vi "Main.InitializeXNET.vi"(7 "Name":string, 8 "error in (no error)":errorcluster, 10 "Data Settings":T12 {"MonitorTool"."Data"."Outgoing"."Trigger.Refs"."Data Reference" format="%.0x"; "MonitorTool"."Data"."Outgoing"."Disable.Refs"."Data Reference" format="%.0x"; "MonitorTool"."Data"."Outgoing"."Data.Refs"."Data Reference" format="%.0x"; "MonitorTool"."Data"."Incoming"."Timing.Refs"."Data Reference" format="%.0x"; "MonitorTool"."Data"."Incoming"."Data.Refs"."Data Reference" format="%.0x"; "MonitorTool"."Network"."Name" format="%.0x"; "SimNodes"."DTCs"."DM1 Ref"."Data Reference" format="%.0x"; "SimNodes"."DTCs"."DM1 Enable Ref"."Data Reference" format="%.0x"; "SimNodes"."DTCs"."DM2 Ref"."Data Reference" format="%.0x"; "SimNodes"."DTCs"."DM2 Enable Ref"."Data Reference" format="%.0x"; "SimNodes"."Network"."Name" format="%.0x"}, 11 "XNET Settings":T2 {"Termination" items=["Off", "On"]}) -> (0 "error out":errorcluster, 3 "Protocol App":T1={"XNET Settings"={"Database"="", "Cluster"="", "Port"="", "Baud rate [Bd]"=0, "Termination"=0, "Incoming Rate"=0, "Outcoming Rate"=1, "Write Decimation"=1}, "Data"=[], "DTCs"=[], "Sim Addresses LUT"=variant, "Data Table LUT"=variant, "MonitorTool.Network"={"Address"=0, "Name"=0}, "Name"=""} {"MonitorTool.Network"."Name" format="%.0x"; "DTCs"."Data"."DM1 Ref"."Data Reference" format="%.0x"; "DTCs"."Data"."DM1 Enable Ref"."Data Reference" format="%.0x"; "DTCs"."Data"."DM2 Ref"."Data Reference" format="%.0x"; "DTCs"."Data"."DM2 Enable Ref"."Data Reference" format="%.0x"; "Data"."Trigger.Refs"."Data Reference" format="%.0x"; "Data"."Disable.Refs"."Data Reference" format="%.0x"; "Data"."Timing.Refs"."Data Reference" format="%.0x"; "Data"."Network"."Name" format="%.0x"; "Data"."IncomingRefs"."Data Reference" format="%.0x"; "Data"."OutgoingRefs"."Data Reference" format="%.0x"; "XNET Settings"."Termination" items=["Off", "On"]})   [LabVIEW 2015, in "J1939 Addon Engine.lvlib"]
uses:
  J1939 Addon Engine.lvlib
  Shared/Types/XNET Settings.ctl
  Shared/Types/Compiled.Node Settings.ctl
  Shared/Types/Compiled Monitor Tool Settings.ctl
  Shared/Types/Monitor Settings.ctl
  Shared/Types/Device Settings.ctl
  Shared/Types/Incoming Settings.ctl
  Shared/Types/Frame Settings.ctl
  Shared/Types/Outgoing Event Trigger Types.ctl
  <vilib>/NI Veristand/Custom Device API/Block Data Reference.ctl
  <vilib>/NI Veristand/Custom Device API/Data Reference.ctl
  Shared/Types/Outgoing Settings.ctl
  Shared/Types/Complied Simulated Device Settings.ctl
  Shared/Types/Compiled Simulated Settings.ctl
  Types/Protocol.App Settings.ctl
  Types/Protocol.XNET Refs.ctl
  Types/Main.Outgoing.Frame.Settings.ctl
  Types/Engine.DTC Settings.ctl
  Types/Engine.DTC FIFOs.ctl
  Types/Engine.Node DTC Settings.ctl
  Shared/J1939 Addon Shared.lvlib
  <vilib>/NI VeriStand/Custom Device API/Custom Device API.lvlib
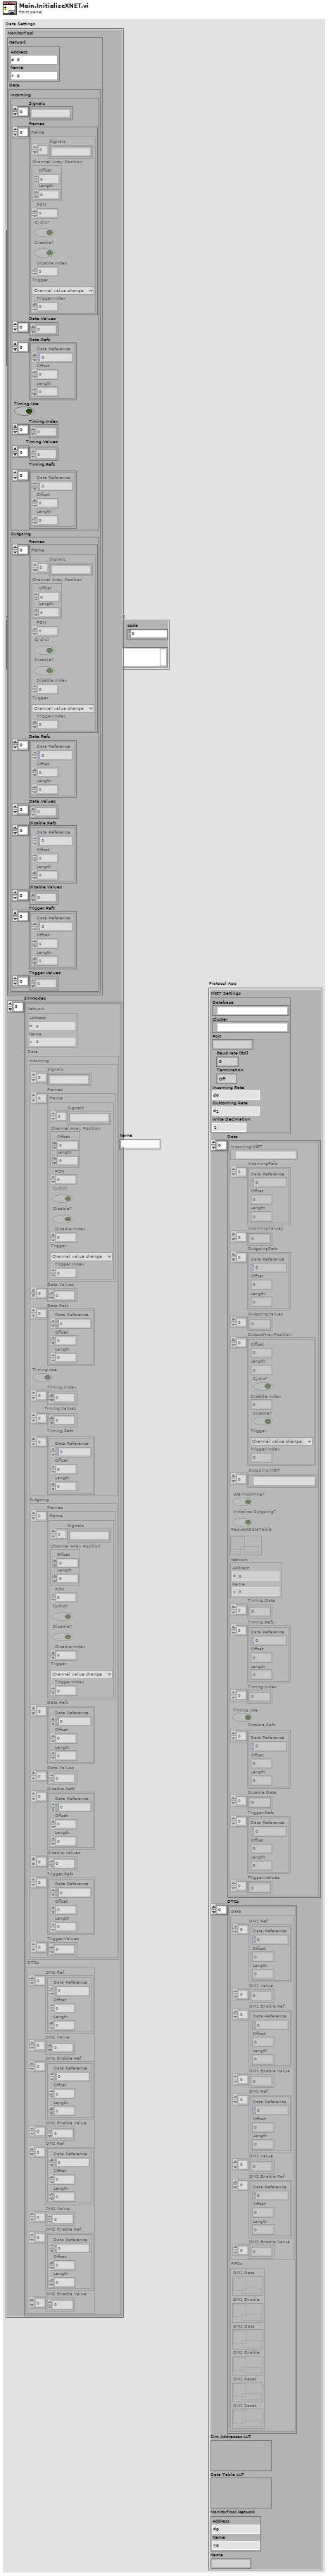
[diagram p1: front panel]
types:
  T1 = typedef "J1939 Addon Engine.lvlib/Protocol.App Settings.ctl" = cluster{"XNET Settings":T2, "Data":T3[], "DTCs":T9[], "Sim Addresses LUT":variant, "Data Table LUT":variant, "MonitorTool.Network":T8, "Name":string}
  T2 = typedef "J1939 Addon Shared.lvlib/XNET Settings.ctl" = cluster{"Database":refnum<k21>, "Cluster":refnum<k21>, "Port":string, "Baud rate [Bd]":u32, "Termination":u32, "Incoming Rate":u32, "Outcoming Rate":u32, "Write Decimation":u32}
  T3 = typedef "J1939 Addon Engine.lvlib/Protocol.XNET Refs.ctl" = cluster{"IncomingXNET":refnum<k21>, "IncomingRefs":T4[], "IncomingValues":dbl[], "OutgoingRefs":T4[], "OutgoingValues":dbl[], "OutputArrayPosition":T6[], "OutgoingXNET":refnum<k21>[], "Use Incoming?":bool, "Initialize Outgoing?":bool, "RequestDataTable":refnum<k33>, "Network":T8, "Timing.Data":dbl[], "Timing.Refs":T4[], "Timing.Index":i32[], "Timing.Use":bool, "Disable.Refs":T4[], "Disable.Data":dbl[], "Trigger.Refs":T4[], "Trigger.Values":dbl[]}
  T4 = typedef "Custom Device API.lvlib/Block Data Reference.ctl" = cluster{"Data Reference":T5, "Offset":u64, "Length":u64}
  T5 = typedef "Custom Device API.lvlib/Data Reference.ctl" = i32
  T6 = typedef "J1939 Addon Engine.lvlib/Main.Outgoing.Frame.Settings.ctl" = cluster{"Offset":u32, "Length":u32, "Cyclic?":bool, "Disable.Index":i32, "Disable?":bool, "Trigger":T7, "Trigger.Index":i32}
  T7 = typedef "J1939 Addon Shared.lvlib/Outgoing Event Trigger Types.ctl" = enum16{"Channel value change", "Trigger channel (not zero)", "Channel value change or trigger channel (not zero)", "Trigger channel (any value change)", "Channel value change or trigger channel (any value change)"}
  T8 = typedef "J1939 Addon Shared.lvlib/Monitor Settings.ctl" = cluster{"Address":u8, "Name":u64}
  T9 = typedef "J1939 Addon Engine.lvlib/Engine.DTC Settings.ctl" = cluster{"Data":T10, "FIFOs":T11}
  T10 = typedef "J1939 Addon Shared.lvlib/Compiled Simulated Settings.ctl" = cluster{"DM1 Ref":T4[], "DM1 Value":dbl[], "DM1 Enable Ref":T4[], "DM1 Enable Value":dbl[], "DM2 Ref":T4[], "DM2 Value":dbl[], "DM2 Enable Ref":T4[], "DM2 Enable Value":dbl[]}
  T11 = typedef "J1939 Addon Engine.lvlib/Engine.DTC FIFOs.ctl" = cluster{"DM1 Data":refnum<k33>, "DM1 Enable":refnum<k33>, "DM2 Data":refnum<k33>, "DM2 Enable":refnum<k33>, "DM1 Reset":refnum<k33>, "DM2 Reset":refnum<k33>}
  T12 = typedef "J1939 Addon Shared.lvlib/Compiled.Node Settings.ctl" = cluster{"MonitorTool":T13, "SimNodes":T18[]}
  T13 = typedef "J1939 Addon Shared.lvlib/Compiled Monitor Tool Settings.ctl" = cluster{"Network":T8, "Data":T14}
  T14 = typedef "J1939 Addon Shared.lvlib/Device Settings.ctl" = cluster{"Incoming":T15, "Outgoing":T17}
  T15 = typedef "J1939 Addon Shared.lvlib/Incoming Settings.ctl" = cluster{"Signals":string[], "Frames":T16[], "Data.Values":dbl[], "Data.Refs":T4[], "Timing.Use":bool, "Timing.Index":i32[], "Timing.Values":dbl[], "Timing.Refs":T4[]}
  T16 = typedef "J1939 Addon Shared.lvlib/Frame Settings.ctl" = cluster{"Signals":string[], "Channel Array Position":cluster{"Offset":u32, "Length":u32}, "PGN":u32, "Cyclic?":bool, "Disable?":bool, "Disable.Index":i32, "Trigger":T7, "Trigger.Index":i32}
  T17 = typedef "J1939 Addon Shared.lvlib/Outgoing Settings.ctl" = cluster{"Frames":T16[], "Data.Refs":T4[], "Data.Values":dbl[], "Disable.Refs":T4[], "Disable.Values":dbl[], "Trigger.Refs":T4[], "Trigger.Values":dbl[]}
  T18 = typedef "J1939 Addon Shared.lvlib/Complied Simulated Device Settings.ctl" = cluster{"Network":T8, "Data":T14, "DTCs":T10}
  T19 = typedef "J1939 Addon Engine.lvlib/Engine.Node DTC Settings.ctl" = cluster{"Network":T8, "Sim DTC Refs":T9}
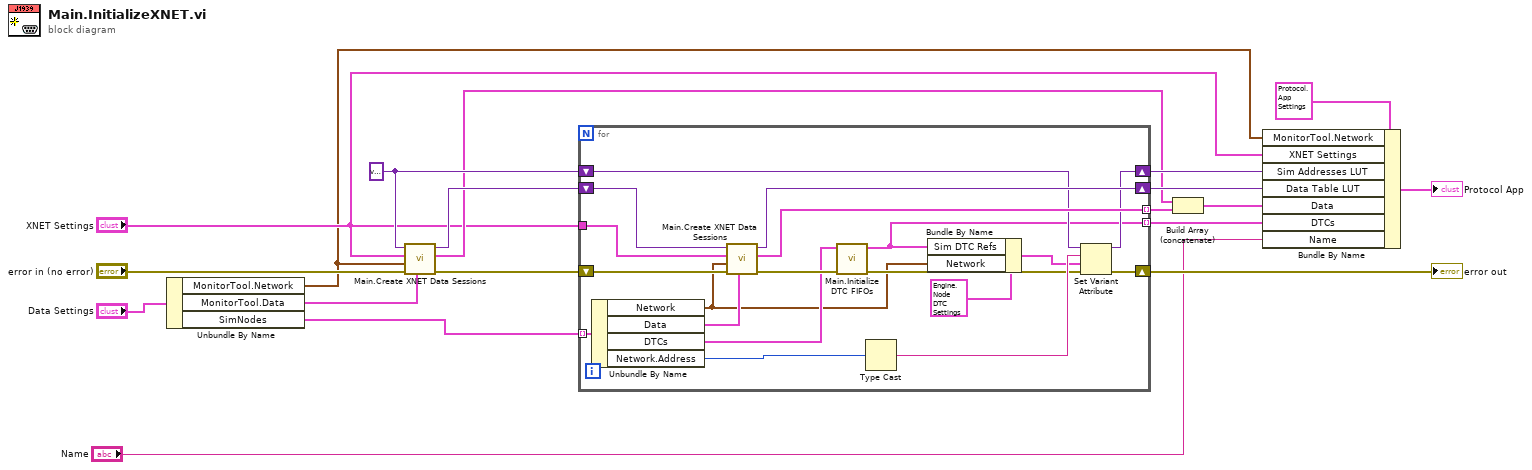
[diagram p0: block diagram]
diagram:
  w14 = variant ("variant")
  n1 = Unbundle By Name("Data Settings") -> ("MonitorTool.Network"=w1:T8, "MonitorTool.Data"=w12:T14, "SimNodes"=w17:T18[])
  n2 = call "Main.Create XNET Data Sessions.vi"("Data"=w12, "error in (no error)"="error in (no error)", "Network"=w1, "J1939 XNET Settings"="XNET Settings", "DataTableLUT"=w14) -> ("error out"=w4:errorcluster, "XNET Sessions"=w5:T3, "DataTableLUT"=w13:variant)  [unwired: 4 in]
  n3 = for {
    tunnel: w17 -> [w34] mode=indexing
    tunnel: "XNET Settings" -> [w35]
    shift-right: [w26] -> w16
    shift-left: w4 -> [w38]
    tunnel: [w37] -> w19 mode=indexing
    shift-right: [w28] -> w8
    shift-left: w13 -> [w32]
    shift-right: [w24] -> w7
    shift-left: w14 -> [w25]
    tunnel: [w23] -> w9 mode=indexing
    n4 = Unbundle By Name(w34) -> ("Network"=w20:T8, "Data"=w33:T14, "DTCs"=w31:T10, "Network.Address"=w29:u8)
    n5 = call "Main.Create XNET Data Sessions.vi"("Data"=w33, "error in (no error)"=w38, "Network"=w20, "J1939 XNET Settings"=w35, "DataTableLUT"=w32) -> ("error out"=w36:errorcluster, "XNET Sessions"=w37:T3, "DataTableLUT"=w28:variant)  [unwired: 4 in]
    n6 = call "Main.Initialize DTC FIFOs.vi"("error in"=w36, "Sim DTCs"=w31) -> ("error out"=w27:errorcluster, "Sim DTC Refs"=w23:T9)  [unwired: 8 in]
    n7 = Type Cast(x=w29) -> (*(type *) &x=w30:string)  [unwired: 1 in]
    n8 = Bundle By Name(cluster=T19 {"Network"={"Address"=0, "Name"=0}, "Sim DTC Refs"={"Data"={"DM1 Ref"=[], "DM1 Value"=[], "DM1 Enable Ref"=[], "DM1 Enable Value"=[], "DM2 Ref"=[], "DM2 Value"=[], "DM2 Enable Ref"=[], "DM2 Enable Value"=[]}, "FIFOs"={"DM1 Data"=refnum, "DM1 Enable"=refnum, "DM2 Data"=refnum, "DM2 Enable"=refnum, "DM1 Reset"=refnum, "DM2 Reset"=refnum}}}, "Sim DTC Refs"=w23, "Network"=w20) -> (w22:T19)
    n9 = Set Variant Attribute(Variant=w25, name=w30, value=w22, error in=w27) -> (Variant out=w24:variant, error out=w26:errorcluster)  [unwired: 1 out]
  }
  "error out" <- w16
  n10 = Build Array (concatenate)(w5, w19) -> (w10:T3[])
  n11 = Bundle By Name(cluster=T1 {"XNET Settings"={"Database"="", "Cluster"="", "Port"="", "Baud rate [Bd]"=0, "Termination"=0, "Incoming Rate"=0, "Outcoming Rate"=1, "Write Decimation"=1}, "Data"=[], "DTCs"=[], "Sim Addresses LUT"=variant, "Data Table LUT"=variant, "MonitorTool.Network"={"Address"=0, "Name"=0}, "Name"=""} ("Protocol App"), "MonitorTool.Network"=w1, "XNET Settings"="XNET Settings", "Sim Addresses LUT"=w7, "Data Table LUT"=w8, "Data"=w10, "DTCs"=w9, "Name"="Name") -> (→"Protocol App":T1)
